vi "Parse Error Log.vi"(10 "Index Timestamp":u64=1724348542139323000, 11 "Error Log":string) -> (3 "Errors":T1[](array[typedef]))   [LabVIEW 2021, in "CIFLogs.lvlib"]
uses:
  CIFLogs.lvlib
  Typedef/Error Message.ctl
panel:
  out "Array":string[](array[string])
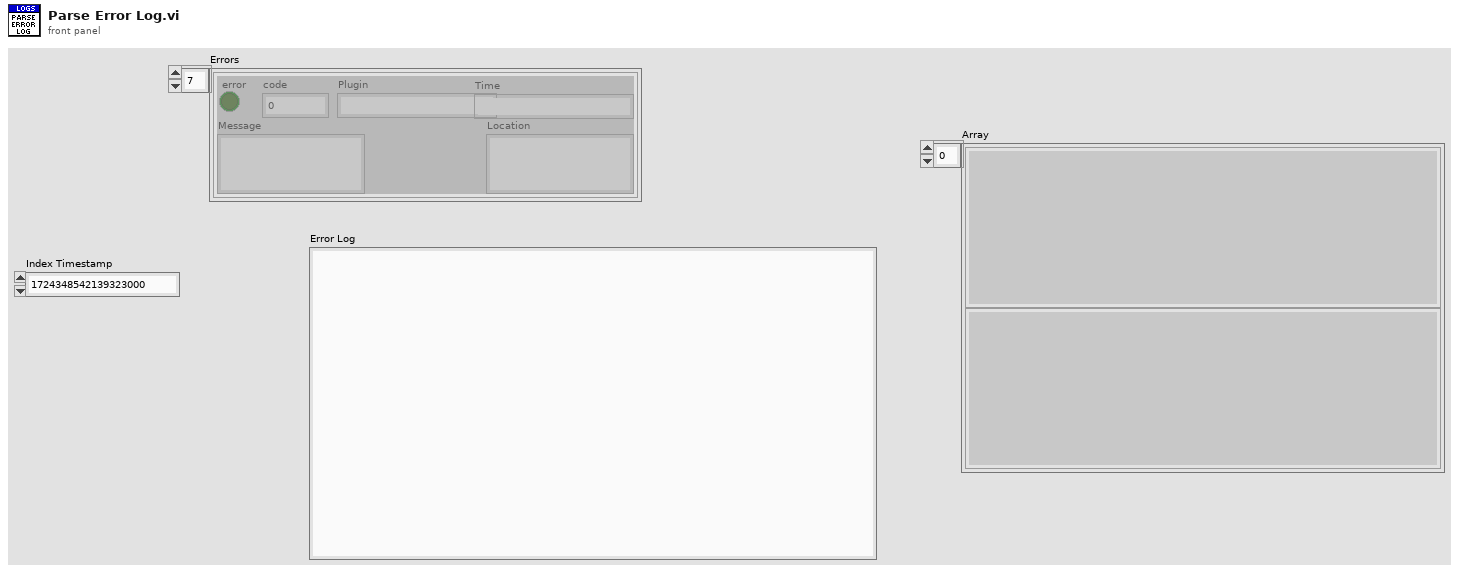
[diagram p1: front panel]
types:
  T1 = typedef "CIFLogs.lvlib/Error Message.ctl" = cluster{"error":bool, "code":i32, "Message":string, "Location":string, "Plugin":string, "Time":string}
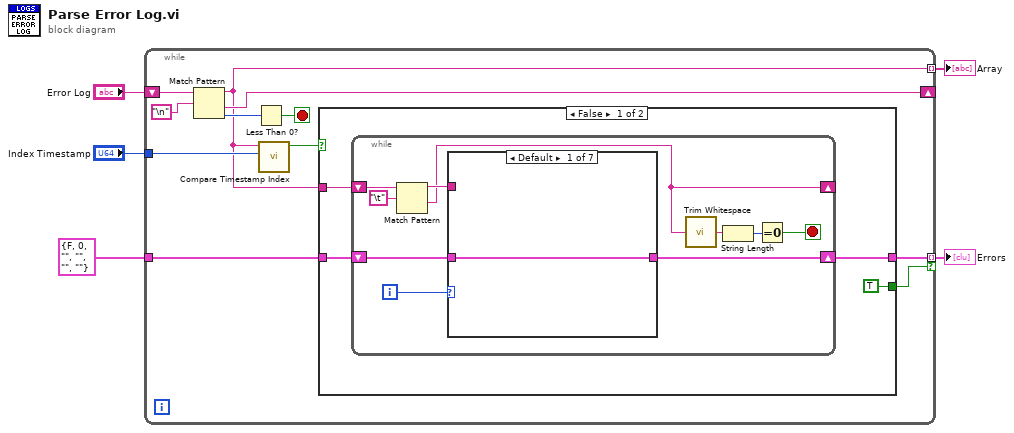
[diagram p0: block diagram]
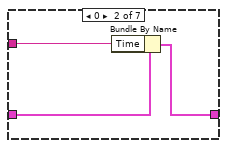
[diagram p2: hidden frame]
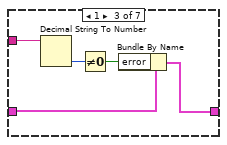
[diagram p3: hidden frame]
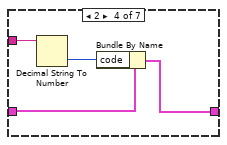
[diagram p4: hidden frame]
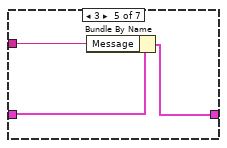
[diagram p5: hidden frame]
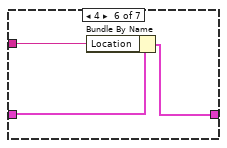
[diagram p6: hidden frame]
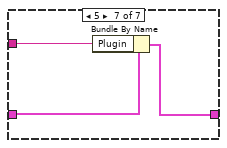
[diagram p7: hidden frame]
diagram:
  n1 = while {
    shift-right: [w14] -> _
    shift-left: "Error Log" -> [w16]
    tunnel: "Index Timestamp" -> [w11]
    tunnel: T1 {"error"=FALSE, "code"=0, "Message"="", "Location"="", "Plugin"="", "Time"=""} ("Error Message") -> [w9]
    tunnel: [w8] -> w4 mode=indexing if=w7
    tunnel: [w6] -> w1 mode=indexing
    stop <- w12 stop-if-true
    n2 = Match Pattern(string=w16, regular expression="\n") -> (before substring=w6:string, after substring=w14:string, offset past match=w13:i32)  [unwired: 1 in, 1 out]
    n3 = Less Than 0?(x=w13) -> (x < 0?=w12:bool)
    n4 = call "Compare Timestamp Index.vi"("Index Timestamp"=w11, "Log Timestamp"=w6) -> ("Past"=w10:bool)  [unwired: 9 in]
    n5 = case shown="False" w10 {
      tunnel: w6 -> [w20 _]
      tunnel: w9 -> [w19 _]
      tunnel: [w18 _] -> w8
      tunnel: [TRUE _] -> w7
      frame False {
        n6 = while {
          shift-right: [w24] -> _
          shift-left: w20 -> [w30]
          shift-right: [w25] -> w18
          shift-left: w19 -> [w26]
          i -> [w28]
          stop <- w21 stop-if-true
          n7 = Match Pattern(string=w30, regular expression="\t") -> (before substring=w27:string, after substring=w24:string)  [unwired: 1 in, 2 out]
          n8 = case shown="Default" w28 {
            tunnel: w27 -> [_ w34 w37 w41 w45 w48 w51]
            tunnel: w26 -> [w31 w33 w39 w43 w46 w49 w52]
            tunnel: [w31 w32 w38 w42 w44 w47 w50] -> w25
            frame Default {
            }
            frame 0 {
              n9 = Bundle By Name(cluster=w33, "Time"=w34) -> (w32:T1)
            }
            frame 1 {
              n10 = Decimal String To Number(string=w37) -> (number=w36:i32)  [unwired: 2 in, 1 out]
              n11 = Not Equal To 0?(x=w36) -> (x != 0?=w35:bool)
              n12 = Bundle By Name(cluster=w39, "error"=w35) -> (w38:T1)
            }
            frame 2 {
              n13 = Decimal String To Number(string=w41) -> (number=w40:i32)  [unwired: 2 in, 1 out]
              n14 = Bundle By Name(cluster=w43, "code"=w40) -> (w42:T1)
            }
            frame 3 {
              n15 = Bundle By Name(cluster=w46, "Message"=w45) -> (w44:T1)
            }
            frame 4 {
              n16 = Bundle By Name(cluster=w49, "Location"=w48) -> (w47:T1)
            }
            frame 5 {
              n17 = Bundle By Name(cluster=w52, "Plugin"=w51) -> (w50:T1)
            }
          }
          n18 = call <vilib>:"Trim Whitespace.vi"("string"=w24) -> ("trimmed string"=w23:string)  [unwired: 1 in]
          n19 = String Length(string=w23) -> (length=w22:i32)
          n20 = Equal To 0?(x=w22) -> (x = 0?=w21:bool)
        }
      }
      frame True {
      }
    }
  }
  "Errors" <- w4
  "Array" <- w1
